vi "Send Settings.vi"(8 "error in":errorcluster, 11 "BKPrecision in":refnum<class "9115AT.lvclass">) -> (0 "error out":errorcluster, 3 "BKPrecision out":refnum<class "9115AT.lvclass">)   [LabVIEW 2018, in "9115AT.lvlib" / "9115AT.lvclass"]
uses:
  9115AT.lvclass
  <instrlib>/BK Precision 911X Series/BK Precision 911X Series.lvlib
  builds/Power_Supply.lvlibp/Power Supply.lvclass
  C:/Users/Ron.Dexter.LUMINARTECH/Desktop/builds/Power_Supply.lvlibp/Power Supply.lvclass
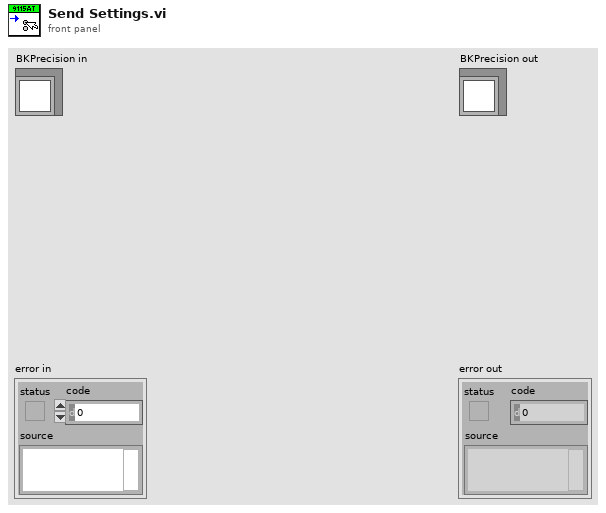
[diagram p1: front panel]
types:
  T1 = typedef "Power_Supply.lvlibp/Supply Settings.ctl" = cluster{"Voltage":dbl, "Current":dbl, "Output":bool}
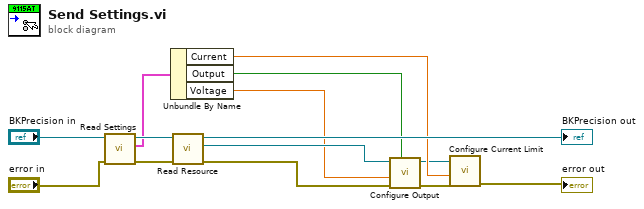
[diagram p0: block diagram]
diagram:
  n1 = call "Read Settings.vi"("error in (no error)"="error in", "Power Supply in"="BKPrecision in") -> ("error out"=w12:errorcluster, "Settings"=w7:T1, "Power Supply out"=w11:refnum<class "9115AT.lvclass">)  [unwired: 7 in]
  n2 = Unbundle By Name(w7) -> ("Current"=w2:dbl, "Output"=w6:bool, "Voltage"=w5:dbl)
  n3 = call "Read Resource.vi"("error in"=w12, "Power Supply in"=w11) -> ("error out"=w8:errorcluster, "Resource"=w9:refnum<visa-resource-name>, "Power Supply out"=→"BKPrecision out":refnum<class "9115AT.lvclass">)  [unwired: 7 in]
  n4 = call <instrlib>:"Configure Output.vi"("Enable Output (T: Enable)"=w6, "error in (no error)"=w8, "Voltage Level (0.0 V)"=w5, "VISA resource name"=w9) -> ("error out"=w4:errorcluster, "VISA resource name out"=w1:refnum<visa-resource-name>)  [unwired: 6 in]
  n5 = call <instrlib>:"Configure Current Limit.vi"("error in (no error)"=w4, "Current Limit (0.0 A)"=w2, "VISA resource name"=w1) -> ("error out"=→"error out":errorcluster)  [unwired: 7 in, 1 out]
